vi "Wait on Listener.vi"(8 "error in":errorcluster, 10 "timeout ms (wait forever: -1)":i32, 11 "TCP slave in":refnum<class "TCP Slave.lvclass">) -> (0 "error out":errorcluster, 1 "Timed Out":bool, 2 "connection reference":refnum<data-value>, 3 "TCP slave out":refnum<class "TCP Slave.lvclass">)   [LabVIEW 2021, in "TCP Slave.lvclass"]
doc: "Wrapper for the wait on listener VI, using the listener stored in the slave and an infinite timeout. When a connection is established, the output class will contain the new connection."
uses:
  TCP Slave.lvclass
  TCP Slave.lvclass/TCP Slave.ctl
  Connection.ctl
  Transmission Data Unit/IP/IP Data Unit.lvclass
  Network Slave.lvclass
  C:/my_projects/projects/Algorithms/Labview/21/Modbus_v121c/Network Protocol/Network Slave/Network Slave.lvclass
  C:/my_projects/projects/Algorithms/Labview/21/Modbus_v121c/Network Protocol/Network Protocol.lvclass
  C:/my_projects/projects/Algorithms/Labview/21/Modbus_v121c/Network Protocol/Network Slave/TCP/TCP Slave.lvclass
  C:/my_projects/projects/Algorithms/Labview/21/Modbus_v121c/Transmission Data Unit/Transmission Data Unit.lvclass
  C:/my_projects/projects/Algorithms/Labview/21/Modbus_v121c/Transmission Data Unit/IP/IP Data Unit.lvclass
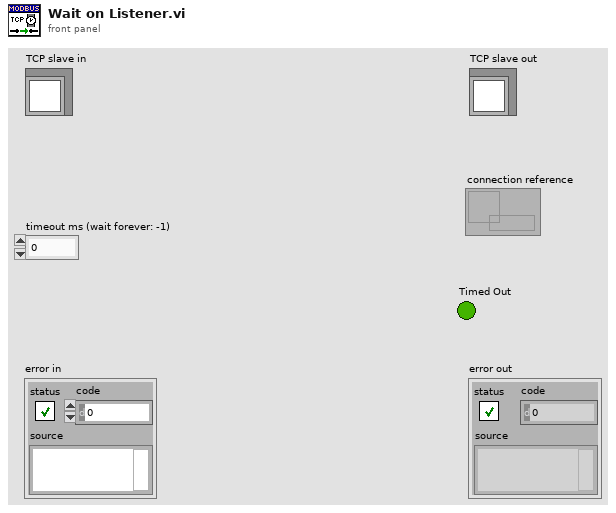
[diagram p1: front panel]
types:
  T1 = typedef "TCP Slave.lvclass/Connection.ctl" = cluster{"Connected?":bool, "IP address":string, "connection error":errorcluster}
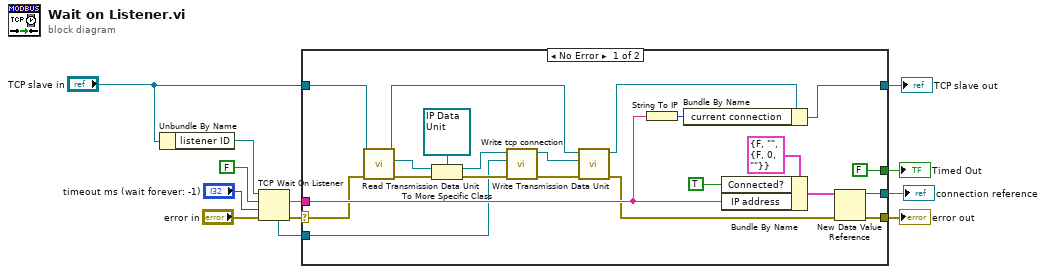
[diagram p0: block diagram]
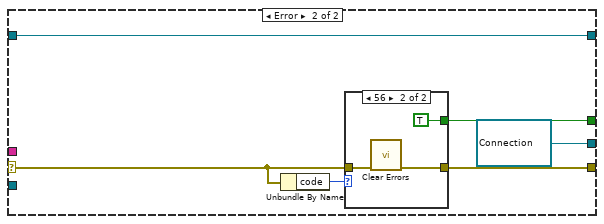
[diagram p2: hidden frame]
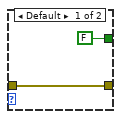
[diagram p3: hidden frame]
diagram:
  n1 = Unbundle By Name("TCP slave in") -> ("listener ID"=w10:refnum<k5>)
  n2 = TCP Wait On Listener(8:"error in", 9:"timeout ms (wait forever: -1)", 10:FALSE ("resolve remote address (T)"), 11:w10) -> (0:w5:errorcluster, 2:w1:string, 4:w9:refnum<k5>)  [unwired: 2 out]
  n3 = case shown="No Error" w5 {
    selector: w5 -> [w20 w39]
    tunnel: "TCP slave in" -> [w26 w36]
    tunnel: w9 -> [w21 _]
    tunnel: [w18 w36] -> w6
    tunnel: [w29 w38] -> w4
    tunnel: [FALSE w37] -> w3
    tunnel: [w33 refnum<data-value> refnum ("data value reference")] -> w2
    tunnel: w1 -> [w28 _]
    frame No Error {
      n4 = call "Read Transmission Data Unit.vi"("error in (no error)"=w20, "Network Slave in"=w26) -> ("error out"=w16:errorcluster, "Transmission Data Unit"=w15:refnum<class "Transmission Data Unit.lvclass">, "Network Slave out"=w25:refnum<class "TCP Slave.lvclass">)  [unwired: 7 in]
      n5 = To More Specific Class(target class=refnum<class "IP Data Unit.lvclass"> refnum ("IP Data Unit"), reference=w15, error in=w16) -> (specific class reference=w23:refnum<class "IP Data Unit.lvclass">, error out=w22:errorcluster)
      n6 = call "Write tcp connection.vi"("error in (no error)"=w22, "tcp connection"=w21, "IP Data Unit in"=w23) -> ("error out"=w14:errorcluster, "IP Data Unit out"=w13:refnum<class "IP Data Unit.lvclass">)  [unwired: 7 in]
      n7 = call "Write Transmission Data Unit.vi"("error in (no error)"=w14, "Transmission Data Unit"=w13, "Network Slave in"=w25) -> ("error out"=w17:errorcluster, "Network Slave out"=w19:refnum<class "TCP Slave.lvclass">)  [unwired: 7 in]
      n8 = String To IP(1:w28) -> (0:w27:u32)
      n9 = Bundle By Name(cluster=w19, "current connection"=w27) -> (w18:refnum<class "TCP Slave.lvclass">)
      n10 = Bundle By Name(cluster=T1 {"Connected?"=FALSE, "IP address"="", "connection error"={"status"=FALSE, "code"=0, "source"=""}} ("Connection"), "Connected?"=TRUE, "IP address"=w28) -> (w31:T1)
      n11 = New Data Value Reference(data value=w31, error in=w17) -> (data value reference=w33:refnum<data-value>, error out=w29:errorcluster)
    }
    frame Error {
      n12 = Unbundle By Name(w39) -> ("code"=w40:i32)
      n13 = case shown="56" w40 {
        tunnel: w39 -> [w42 w45]
        tunnel: [w42 w44] -> w38
        tunnel: [FALSE TRUE] -> w37
        frame Default {
        }
        frame 56 {
          n14 = call <vilib>:"Clear Errors.vi"("error in (no error)"=w45) -> ("error out"=w44:errorcluster)  [unwired: 5 in, 1 out]
        }
      }
    }
  }
  "error out" <- w4
  "Timed Out" <- w3
  "connection reference" <- w2
  "TCP slave out" <- w6
